vi "UI-main.vi"() -> ()   [LabVIEW 2013]
uses:
  <vilib>/LabVIEW Targets/FPGA/cRIO/shared/nicrio_ModuleControls/nicrio_cRIO-9229_DataRatesRing.ctl
  <vilib>/LabVIEW Targets/FPGA/cRIO/shared/nicrio_ModuleControls/nicrio_cRIO-9205_VoltageRange.ctl
  <vilib>/LabVIEW Targets/FPGA/cRIO/shared/nicrio_ModuleControls/nicrio_cRIO-9205_TerminalMode.ctl
panel:
  in  "配置簇":T4={"9205Count(uSec)"=1000, "9229采样率"=25, "update9213"=TRUE, "9213转换时间"=enum."High Speed", "9205Update AI Setings"=TRUE, "9205AI Channel Settings"=[{"Voltage Range"=enum."+/- 10V", "Terminal Mode"=enum."RSE"}, {"Voltage Range"=enum."+/- 10V", "Terminal Mode"=enum."RSE"}, {"Voltage Range"=enum."+/- 10V", "Terminal Mode"=enum."RSE"}, {"Voltage Range"=enum."+/- 10V", "Terminal Mode"=enum."RSE"}, {"Voltage Range"=enum."+/- 10V", "Terminal Mode"=enum."RSE"}, {"Voltage Range"=enum."+/- 10V", "Terminal Mode"=enum."RSE"}, {"Voltage Range"=enum."+/- 10V", "Terminal Mode"=enum."RSE"}, {"Voltage Range"=enum."+/- 10V", "Terminal Mode"=enum."RSE"}, {"Voltage Range"=enum."+/- 10V", "Terminal Mode"=enum."RSE"}, {"Voltage Range"=enum."+/- 10V", "Terminal Mode"=enum."RSE"}, {"Voltage Range"=enum."+/- 10V", "Terminal Mode"=enum."RSE"}, {"Voltage Range"=enum."+/- 10V", "Terminal Mode"=enum."RSE"}, {"Voltage Range"=enum."+/- 10V", "Terminal Mode"=enum."RSE"}, {"Voltage Range"=enum."+/- 10V", "Terminal Mode"=enum."RSE"}, {"Voltage Range"=enum."+/- 10V", "Terminal Mode"=enum."RSE"}, {"Voltage Range"=enum."+/- 10V", "Terminal Mode"=enum."RSE"}, {"Voltage Range"=enum."+/- 10V", "Terminal Mode"=enum."RSE"}, {"Voltage Range"=enum."+/- 10V", "Terminal Mode"=enum."RSE"}, {"Voltage Range"=enum."+/- 10V", "Terminal Mode"=enum."RSE"}, {"Voltage Range"=enum."+/- 10V", "Terminal Mode"=enum."RSE"}, {"Voltage Range"=enum."+/- 10V", "Terminal Mode"=enum."RSE"}, {"Voltage Range"=enum."+/- 10V", "Terminal Mode"=enum."RSE"}, {"Voltage Range"=enum."+/- 10V", "Terminal Mode"=enum."RSE"}, {"Voltage Range"=enum."+/- 10V", "Terminal Mode"=enum."RSE"}, {"Voltage Range"=enum."+/- 10V", "Terminal Mode"=enum."RSE"}]} {"9229采样率" items=["", "50.000 kS/s (NI 9229)", "25.000 kS/s (NI 9229)", "16.667 kS/s (NI 9229)", "12.500 kS/s (NI 9229)", "10.000 kS/s (NI 9229)", "8.333 kS/s (NI 9229)", "7.143 kS/s (NI 9229)", "6.250 kS/s (NI 9229)", "5.556 kS/s (NI 9229)", "5.000 kS/s (NI 9229)", "4.545 kS/s (NI 9229)", "4.167 kS/s (NI 9229)", "3.846 kS/s (NI 9229)", "3.571 kS/s (NI 9229)", "3.333 kS/s (NI 9229)", "3.125 kS/s (NI 9229)", "2.941 kS/s (NI 9229)", "2.778 kS/s (NI 9229)", "2.632 kS/s (NI 9229)", "2.500 kS/s (NI 9229)", "2.381 kS/s (NI 9229)", "2.273 kS/s (NI 9229)", "2.174 kS/s (NI 9229)", "2.083 kS/s (NI 9229)", "2.000 kS/s (NI 9229)", "1.923 kS/s (NI 9229)", "1.852 kS/s (NI 9229)", "1.786 kS/s (NI 9229)", "1.724 kS/s (NI 9229)", "1.667 kS/s (NI 9229)", "1.613 kS/s (NI 9229)"]}
  in  "选项卡控件":T5(tab)=enum."9205电流监控 "
  out "9213数据":T6(graph)={1372.0, 1372.0, 0.0, 0.0, 0.0, 0.0, 0.0, 0.0, 0.0, 0.0, 0.0, 0.0, 0.0, 0.0, 0.0, 0.0}
  out "9213通道1数据":dbl=1372.0
  out "9213通道2数据":dbl=1372.0
  out "9213通道3数据":dbl
  out "9213通道4数据":dbl
  out "9213通道5数据":dbl
  out "9213通道6数据":dbl
  out "9213通道7数据":dbl
  out "9213通道8数据":dbl
  out "9213通道9数据":dbl
  out "9213通道10数据":dbl
  out "9213通道11数据":dbl
  out "9213通道12数据":dbl
  out "9213通道13数据":dbl
  out "9213通道14数据":dbl
  out "9213通道15数据":dbl
  out "9213通道16数据":dbl
  out "9229通道12数据":dbl
  out "9229通道8数据":dbl
  out "9229通道10数据":dbl
  out "9229通道9数据":dbl
  out "9229通道6数据":dbl
  out "9229通道5数据":dbl
  out "9229通道4数据":dbl
  out "9229通道3数据":dbl
  out "9229通道2数据":dbl=24.32616424560547
  out "9229通道1数据":dbl=0.00066375732421875
  out "9229通道7数据":dbl
  out "9229通道11数据":dbl
  out "9229通道13数据":dbl
  out "9229通道14数据":dbl
  out "9229通道15数据":dbl
  out "9229通道16数据":dbl
  out "9229":T6(graph)={0.00066375732421875, 24.32616424560547, 0.0, 0.0, 0.0, 0.0, 0.0, 0.0, 0.0, 0.0, 0.0, 0.0, 0.0, 0.0, 0.0, 0.0}
  out "9205电压通道2":dbl=-3.0960659980773926
  out "9205电压通道1":dbl=-3.097379207611084
  out "9205电压通道3":dbl
  out "9205电压通道4":dbl
  out "9205电压通道5":dbl
  out "9205电压通道6":dbl
  out "9205电压通道7":dbl
  out "9205电压通道8":dbl
  out "9205电压通道9":dbl
  out "9205电压通道10":dbl
  out "9205电压通道11":dbl
  out "9205电压通道12":dbl
  out "9205电压通道13":dbl
  out "9205电压通道14":dbl
  out "9205电压通道15":dbl
  out "9205电压通道16":dbl
  out "9205电压通道17":dbl
  out "9205电压通道18":dbl
  out "9205电压通道19":dbl
  out "9205电压通道20":dbl
  out "9205电压通道21":dbl
  out "9205电压通道22":dbl
  out "9205电压通道23":dbl
  out "9205电压通道24":dbl
  out "9205电压":T7(graph)={-3.097379207611084, -3.0960659980773926, 0.0, 0.0, 0.0, 0.0, 0.0, 0.0, 0.0, 0.0, 0.0, 0.0, 0.0, 0.0, 0.0, 0.0, 0.0, 0.0, 0.0, 0.0, 0.0, 0.0, 0.0, 0.0, 0.0}
  out "9205电压通道25":dbl
  out "9205电流通道2":dbl=-3.0373048782348633
  out "9205电流通道1":dbl=-3.005133628845215
  out "9205电流通道3":dbl
  out "9205电流通道4":dbl
  out "9205电流通道5":dbl
  out "9205电流通道6":dbl
  out "9205电流通道7":dbl
  out "9205电流 2":cluster{dbl, dbl, dbl, dbl, dbl, dbl, dbl}(graph)={-3.005133628845215, -3.0373048782348633, 0.0, 0.0, 0.0, 0.0, 0.0}
  in  "9205电流":string(tree)="2"
  in  "9205电压":string(tree)="2"
  in  "9213温度":string(tree)="2"
  in  "9229电压":string(tree)="2"
  out "连接成功？":bool
  out "UI命令":string="退出"
  in  "停止发送数据到UI":bool
  in  "发送数据到UI":bool
  in  "连接":bool=TRUE
  in  "触发采集":bool=TRUE
  in  "退出":bool=TRUE
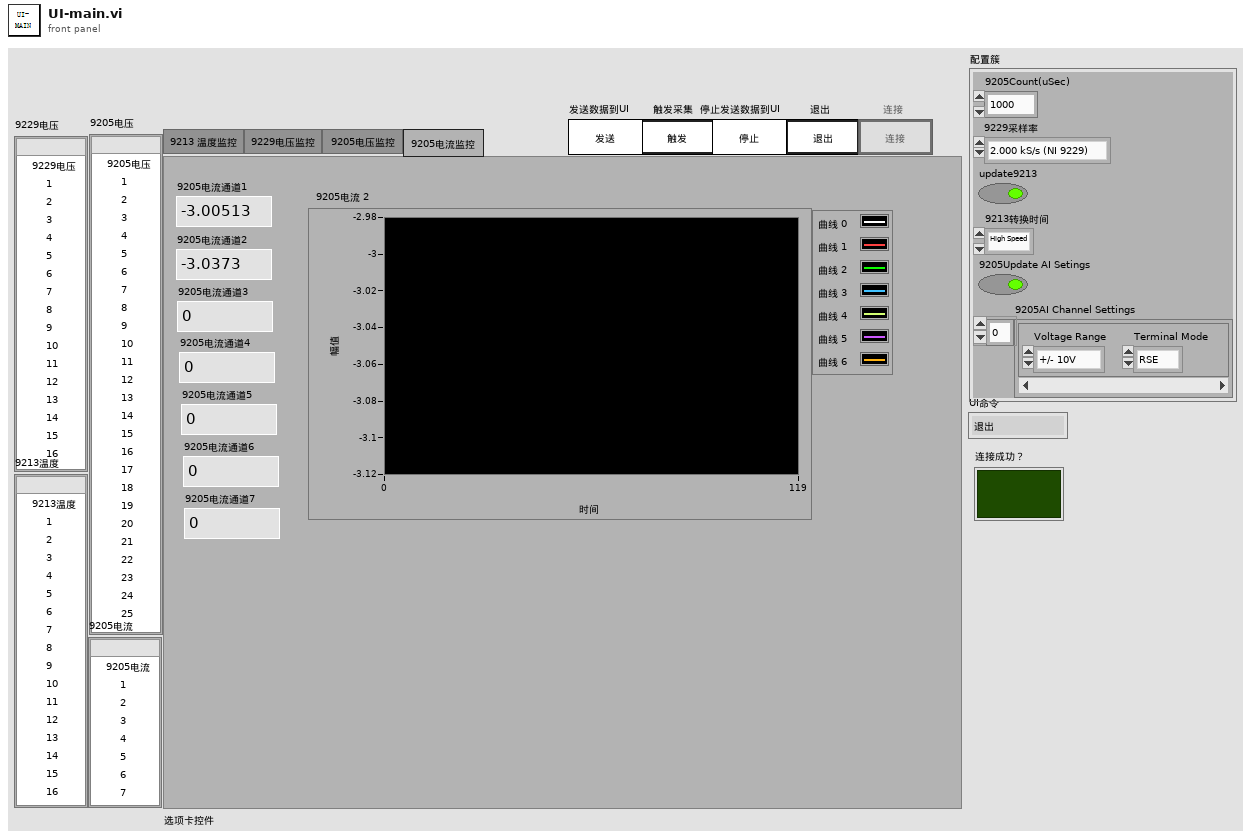
[diagram p1: front panel]
types:
  T1 = typedef "nicrio_cRIO-9229_DataRatesRing.ctl" = u8
  T2 = typedef "nicrio_cRIO-9205_VoltageRange.ctl" = enum8{"+/- 10V", "+/- 5V", "+/- 1V", "+/- 200mV"}
  T3 = typedef "nicrio_cRIO-9205_TerminalMode.ctl" = enum8{"RSE", "NRSE", "DIFF"}
  T4 = cluster{"9205Count(uSec)":u32, "9229采样率":T1, "update9213":bool, "9213转换时间":enum8{"High Speed", "High Resolution"}, "9205Update AI Setings":bool, "9205AI Channel Settings":cluster{"Voltage Range":T2, "Terminal Mode":T3}[]}
  T5 = enum32{"9213 温度监控", "9229电压监控", "9205电压监控 ", "9205电流监控 "}
  T6 = cluster{dbl, dbl, dbl, dbl, dbl, dbl, dbl, dbl, dbl, dbl, dbl, dbl, dbl, dbl, dbl, dbl}
  T7 = cluster{dbl, dbl, dbl, dbl, dbl, dbl, dbl, dbl, dbl, dbl, dbl, dbl, dbl, dbl, dbl, dbl, dbl, dbl, dbl, dbl, dbl, dbl, dbl, dbl, dbl}
  T8 = enum16{"open", "open or create", "create or replace", "create", "open (read-only)"}
  T9 = typedef "消息命令控件.ctl" = cluster{"message":string, "变体数据":variant}
  T10 = typedef "LVPoint32TypeDef.ctl" = cluster{"Horizontal":i32, "Vertical":i32}
  T11 = enum8{"Enabled", "Disabled", "Disabled and Grayed Out"}
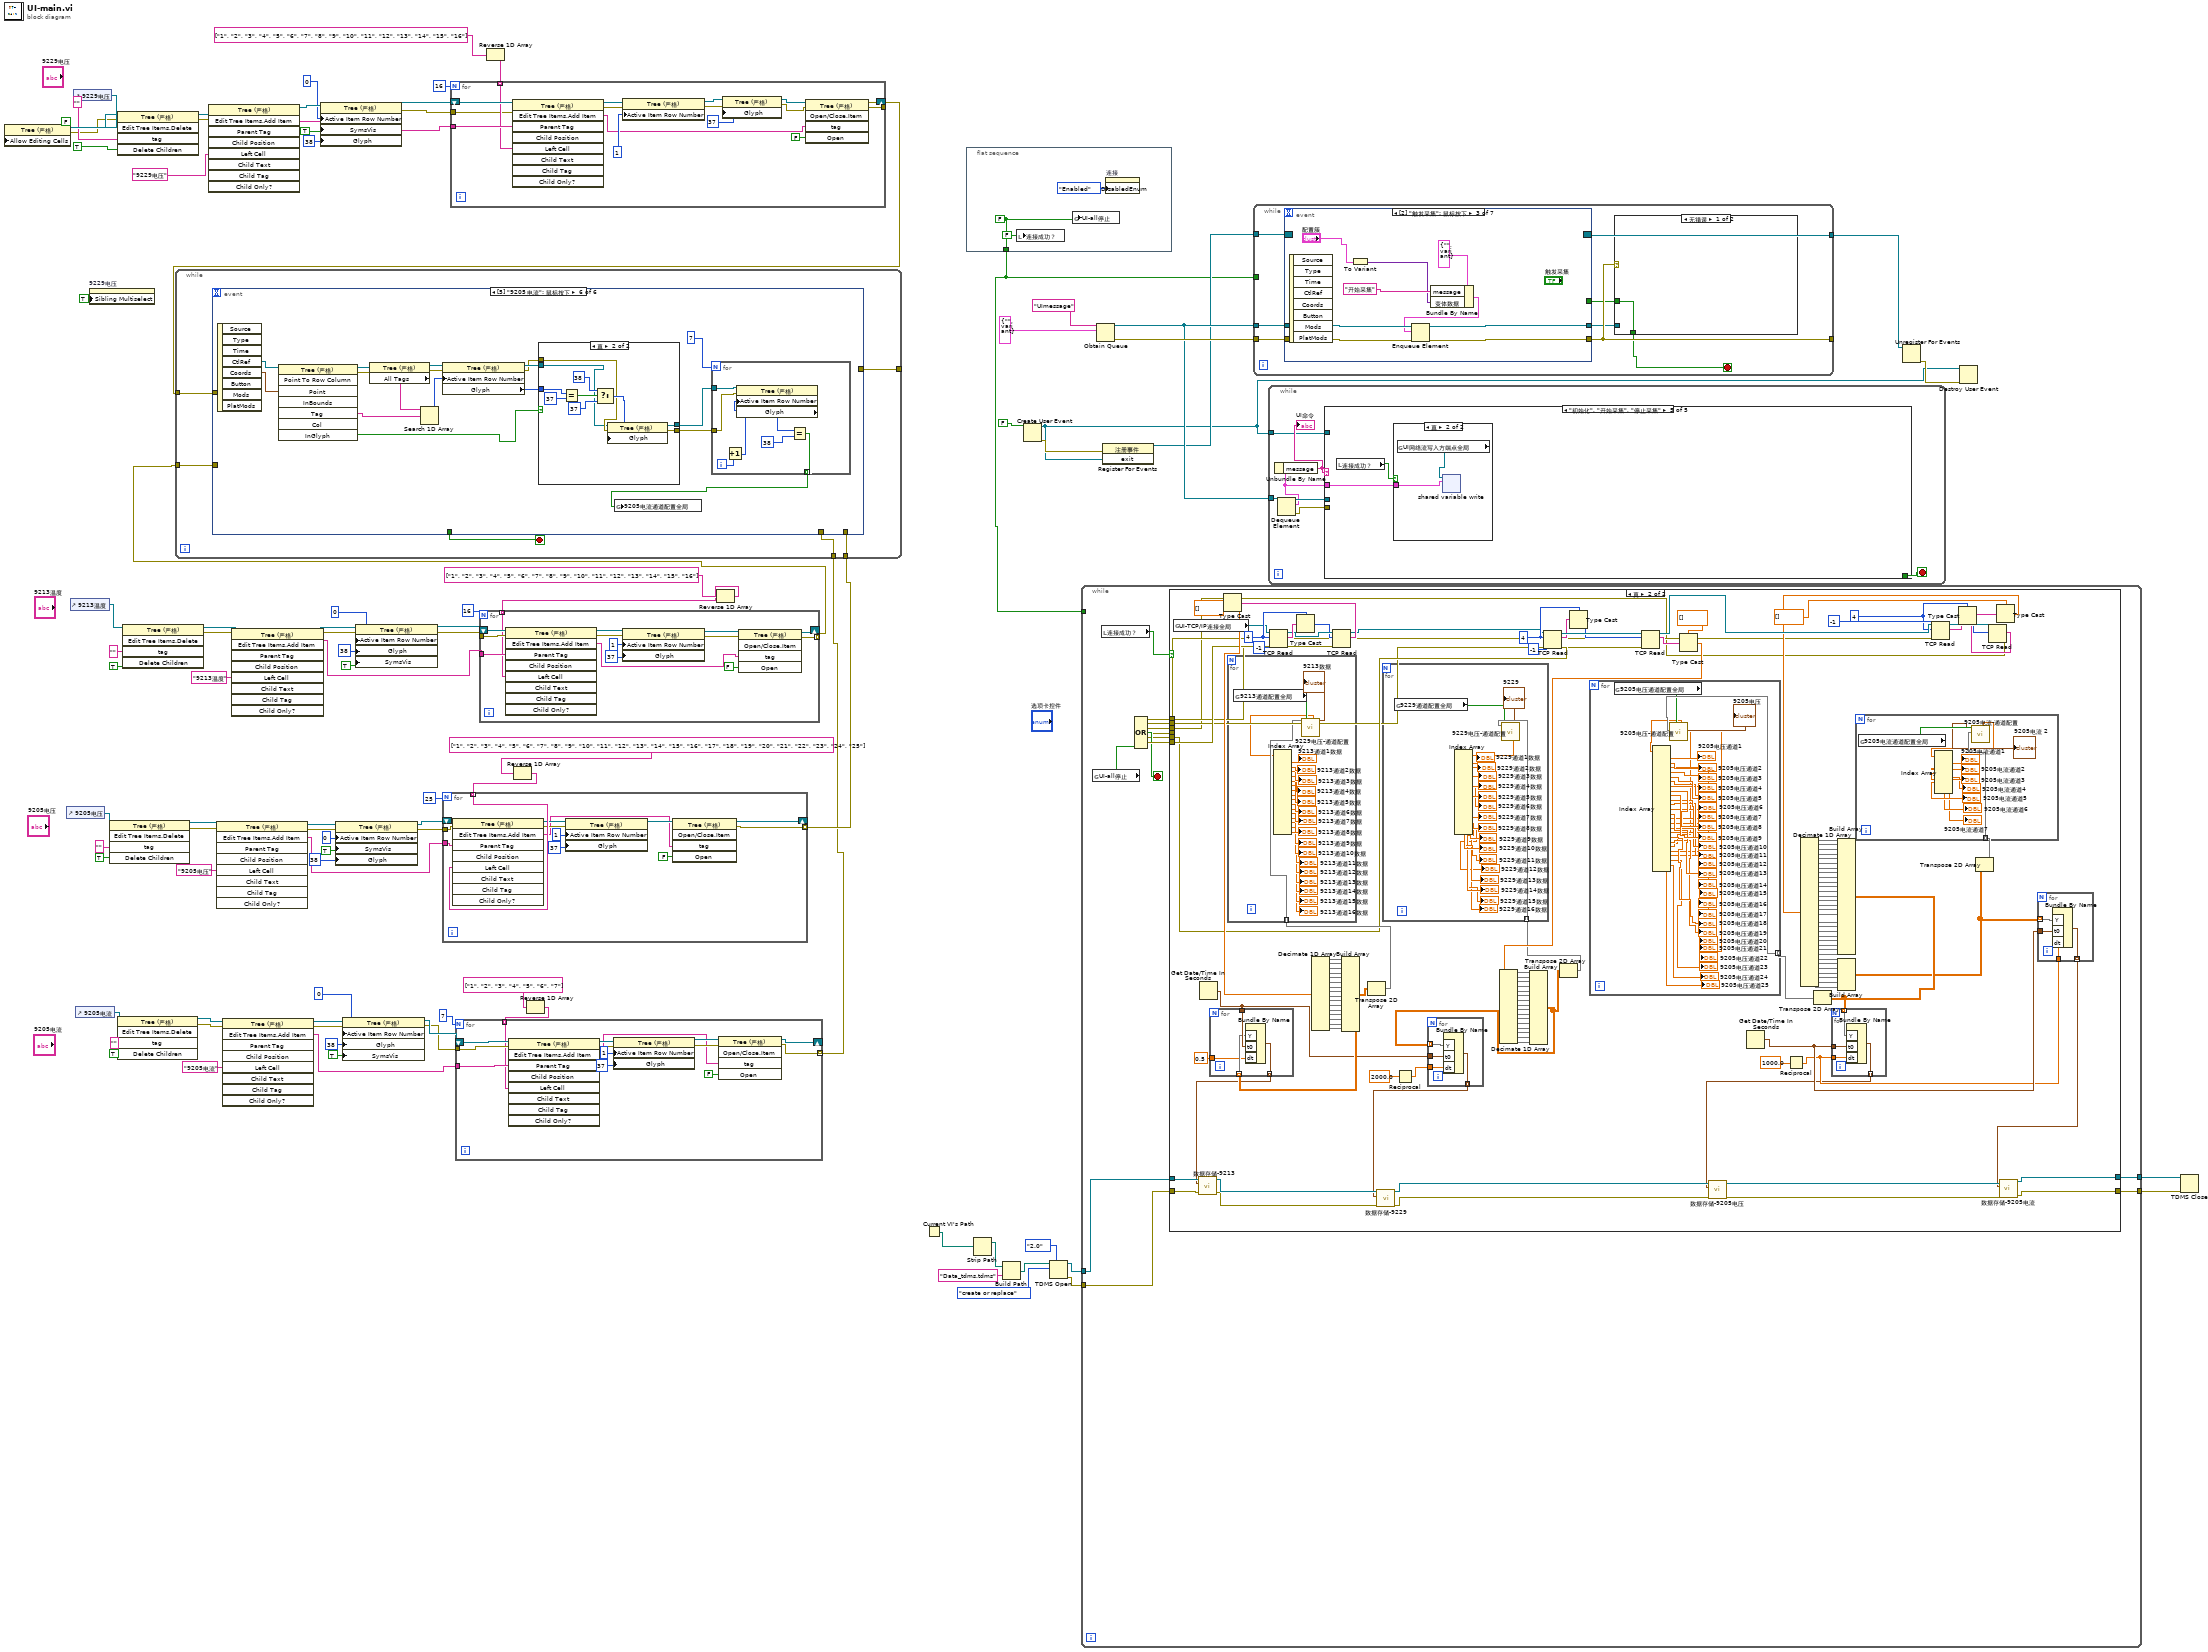
[diagram p0: block diagram]
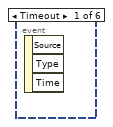
[diagram p2: hidden frame]
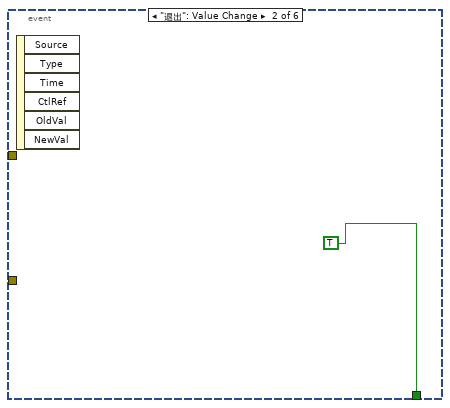
[diagram p3: hidden frame]
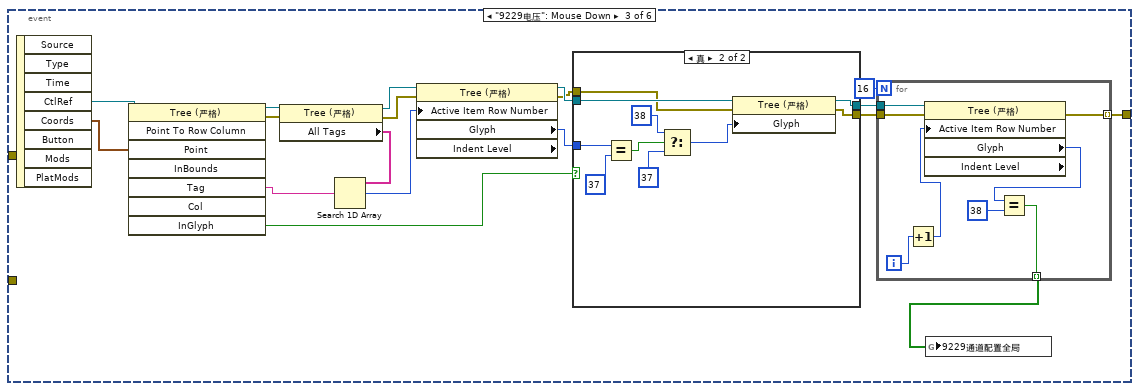
[diagram p4: hidden frame]
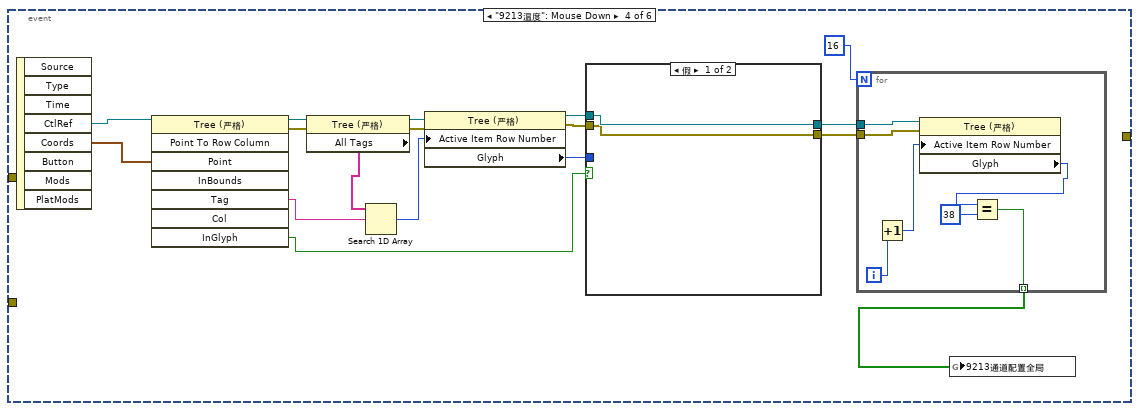
[diagram p6: hidden frame]
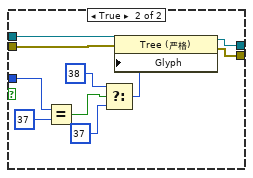
[diagram p7: hidden frame]
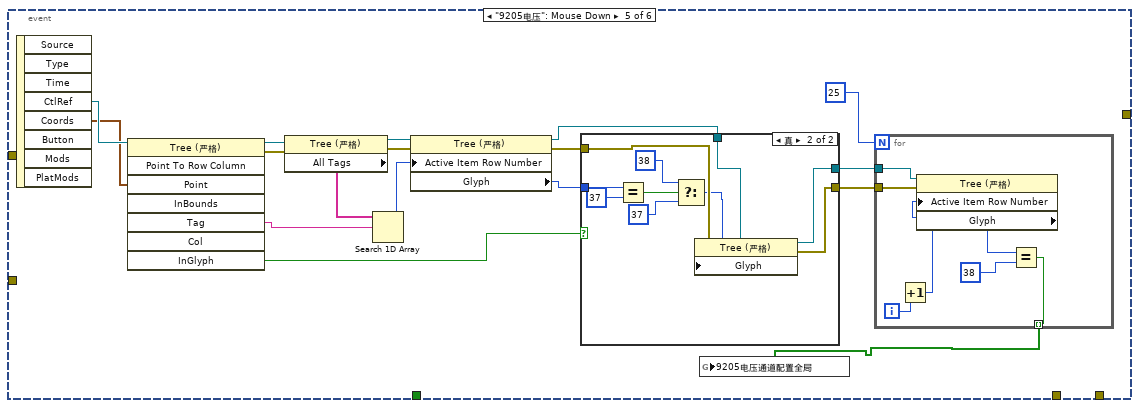
[diagram p8: hidden frame]
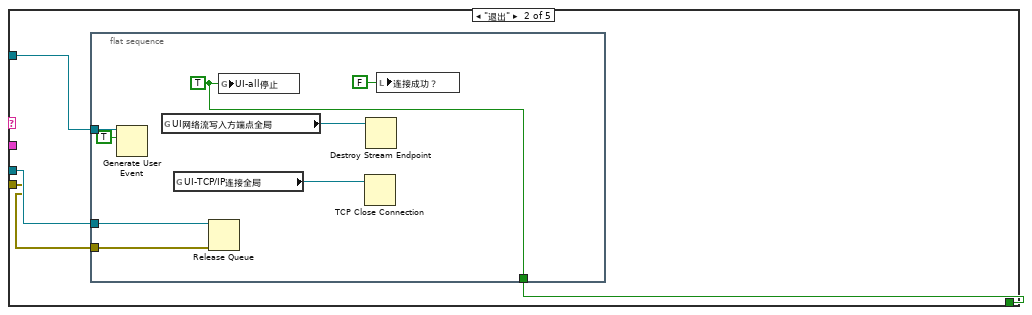
[diagram p13: hidden frame]
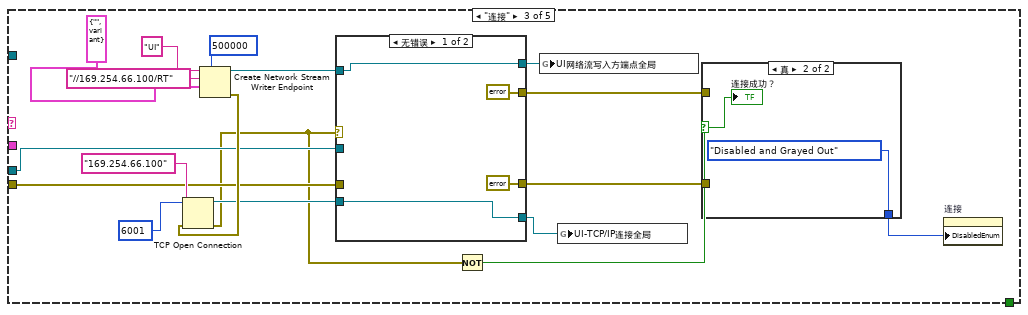
[diagram p14: hidden frame]
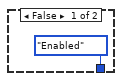
[diagram p15: hidden frame]
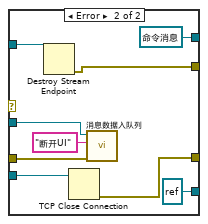
[diagram p16: hidden frame]
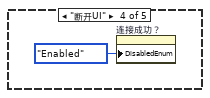
[diagram p17: hidden frame]
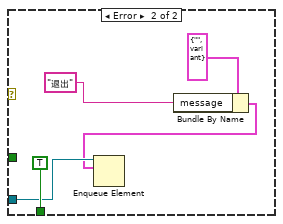
[diagram p19: hidden frame]
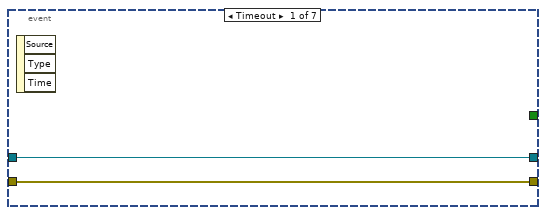
[diagram p20: hidden frame]
diagram:
  n1 = control-ref of="9205电压"() -> (w53:refnum<vi>)
  n2 = control-ref of="9213温度"() -> (w71:refnum<vi>)
  n3 = control-ref of="9229电压"() -> (w91:refnum<vi>)
  n4 = property class="Tree (严格)"(reference=w91, "Allow Editing Cells"=FALSE ("允许编辑单元格")) -> (reference out=w89:refnum<vi>, error out=w84:errorcluster)  [unwired: 1 in]
  n5 = control-ref of="9205电流"() -> (w37:refnum<vi>)
  n6 = property on="9229电压" class="Tree (严格)"("Sibling Multiselect"=TRUE ("同辈多选")) -> ()  [unwired: 2 in, 2 out]
  n7 = invoke class="Tree (严格)" method="Edit Tree Items.Delete"(reference=w53, "tag"="" ("标识符"), "Delete Children"=TRUE ("删除子项？")) -> (reference out=w50:refnum<vi>, error out=w49:errorcluster)  [unwired: 2 in, 3 out]
  n8 = invoke class="Tree (严格)" method="Edit Tree Items.Delete"(reference=w37, "tag"="" ("标识符"), "Delete Children"=TRUE ("删除子项？")) -> (reference out=w34:refnum<vi>, error out=w33:errorcluster)  [unwired: 2 in, 3 out]
  n9 = invoke class="Tree (严格)" method="Edit Tree Items.Delete"(reference=w89, error in=w84, "tag"="" ("标识符"), "Delete Children"=TRUE ("删除子项？")) -> (reference out=w87:refnum<vi>, error out=w83:errorcluster)  [unwired: 1 in, 3 out]
  n10 = invoke class="Tree (严格)" method="Edit Tree Items.Delete"(reference=w71, "tag"="" ("标识符"), "Delete Children"=TRUE ("删除子项？")) -> (reference out=w68:refnum<vi>, error out=w67:errorcluster)  [unwired: 2 in, 3 out]
  n11 = invoke class="Tree (严格)" method="Edit Tree Items.Add Item"(reference=w87, error in=w83, "Left Cell"="9229电压" ("左单元格字符串")) -> (reference out=w81:refnum<vi>, "Edit Tree Items:Add Item"=w73:string)  [unwired: 6 in, 7 out]
  n12 = invoke class="Tree (严格)" method="Edit Tree Items.Add Item"(reference=w50, error in=w49, "Left Cell"="9205电压" ("左单元格字符串")) -> (reference out=w47:refnum<vi>, error out=w46:errorcluster, "Edit Tree Items:Add Item"=w41:string)  [unwired: 6 in, 6 out]
  n13 = invoke class="Tree (严格)" method="Edit Tree Items.Add Item"(reference=w34, error in=w33, "Left Cell"="9205电流" ("左单元格字符串")) -> (reference out=w31:refnum<vi>, error out=w30:errorcluster, "Edit Tree Items:Add Item"=w22:string)  [unwired: 6 in, 6 out]
  n14 = invoke class="Tree (严格)" method="Edit Tree Items.Add Item"(reference=w68, error in=w67, "Left Cell"="9213温度" ("左单元格字符串")) -> (reference out=w65:refnum<vi>, error out=w64:errorcluster, "Edit Tree Items:Add Item"=w56:string)  [unwired: 6 in, 6 out]
  n15 = property class="Tree (严格)"(reference=w81, "Active Item Row Number"=0 ("活动项:行数"), "SymsVis"=TRUE ("显示项:显示符号"), "Glyph"=38 ("活动项:符号索引")) -> (reference out=w77:refnum<vi>, error out=w76:errorcluster)  [unwired: 1 in]
  n16 = property class="Tree (严格)"(reference=w47, error in=w46, "Active Item Row Number"=0 ("活动项:行数"), "SymsVis"=TRUE ("显示项:显示符号"), "Glyph"=38 ("活动项:符号索引")) -> (reference out=w43:refnum<vi>, error out=w42:errorcluster)
  n17 = property class="Tree (严格)"(reference=w31, error in=w30, "Active Item Row Number"=0 ("活动项:行数"), "Glyph"=38 ("活动项:符号索引"), "SymsVis"=TRUE ("显示项:显示符号")) -> (reference out=w24:refnum<vi>, error out=w23:errorcluster)
  n18 = property class="Tree (严格)"(reference=w65, error in=w64, "Active Item Row Number"=0 ("活动项:行数"), "Glyph"=38 ("活动项:符号索引"), "SymsVis"=TRUE ("显示项:显示符号")) -> (reference out=w58:refnum<vi>, error out=w57:errorcluster)
  n19 = Reverse 1D Array(array=string[] ["1", "2", "3", "4", "5", "6", "7", "8", "9", "10", "11", "12", "13", "14", "15", "16"]) -> (reversed array=w79:string[])
  n20 = for {
    N: 16 -> [_]
    tunnel: w73 -> [w112]
    tunnel: w79 -> [w110] mode=indexing
    tunnel: w76 -> [w109]
    tunnel: [w103] -> w72
    shift-right: [w102] -> _
    shift-left: w77 -> [w111]
    n21 = invoke class="Tree (严格)" method="Edit Tree Items.Add Item"(reference=w111, error in=w109, "Parent Tag"=w112, "Left Cell"=w110) -> (reference out=w108:refnum<vi>, error out=w107:errorcluster, "Edit Tree Items:Add Item"=w98:string)  [unwired: 5 in, 6 out]
    n22 = property class="Tree (严格)"(reference=w108, error in=w107, "Active Item Row Number"=1 ("活动项:行数")) -> (reference out=w106:refnum<vi>, error out=w99:errorcluster)
    n23 = property class="Tree (严格)"(reference=w106, error in=w99, "Glyph"=37 ("活动项:符号索引")) -> (reference out=w101:refnum<vi>, error out=w100:errorcluster)
    n24 = invoke class="Tree (严格)" method="Open/Close.Item"(reference=w101, error in=w100, "tag"=w98, "Open"=FALSE ("打开？")) -> (reference out=w102:refnum<vi>, error out=w103:errorcluster)  [unwired: 1 in, 3 out]
  }
  n25 = Reverse 1D Array(array=string[] ["1", "2", "3", "4", "5", "6", "7", "8", "9", "10", "11", "12", "13", "14", "15", "16", "17", "18", "19", "20", "21", "22", "23", "24", "25"]) -> (reversed array=w39:string[])
  n26 = for {
    N: 25 -> [_]
    tunnel: w42 -> [w124]
    shift-right: [w116] -> _
    shift-left: w43 -> [w125]
    tunnel: w41 -> [w123]
    tunnel: w39 -> [w122] mode=indexing
    tunnel: [w113] -> w38 mode=indexing
    n27 = invoke class="Tree (严格)" method="Edit Tree Items.Add Item"(reference=w125, error in=w124, "Parent Tag"=w123, "Left Cell"=w122) -> (reference out=w121:refnum<vi>, error out=w120:errorcluster, "Edit Tree Items:Add Item"=w115:string)  [unwired: 5 in, 6 out]
    n28 = property class="Tree (严格)"(reference=w121, error in=w120, "Active Item Row Number"=1 ("活动项:行数"), "Glyph"=37 ("活动项:符号索引")) -> (reference out=w117:refnum<vi>)  [unwired: 1 out]
    n29 = invoke class="Tree (严格)" method="Open/Close.Item"(reference=w117, "tag"=w115, "Open"=FALSE ("打开？")) -> (reference out=w116:refnum<vi>, error out=w113:errorcluster)  [unwired: 2 in, 3 out]
  }
  n30 = Reverse 1D Array(array=string[] ["1", "2", "3", "4", "5", "6", "7"]) -> (reversed array=w20:string[])
  n31 = for {
    N: 7 -> [_]
    shift-right: [w127] -> _
    shift-left: w24 -> [w139]
    tunnel: w23 -> [w138]
    tunnel: w22 -> [w137]
    tunnel: w20 -> [w136] mode=indexing
    tunnel: [w126] -> w19 mode=indexing
    n32 = invoke class="Tree (严格)" method="Edit Tree Items.Add Item"(reference=w139, error in=w138, "Parent Tag"=w137, "Left Cell"=w136) -> (reference out=w135:refnum<vi>, error out=w134:errorcluster, "Edit Tree Items:Add Item"=w129:string)  [unwired: 5 in, 6 out]
    n33 = property class="Tree (严格)"(reference=w135, error in=w134, "Active Item Row Number"=1 ("活动项:行数"), "Glyph"=37 ("活动项:符号索引")) -> (reference out=w131:refnum<vi>, error out=w130:errorcluster)
    n34 = invoke class="Tree (严格)" method="Open/Close.Item"(reference=w131, error in=w130, "tag"=w129, "Open"=FALSE ("打开？")) -> (reference out=w127:refnum<vi>, error out=w126:errorcluster)  [unwired: 1 in, 3 out]
  }
  n35 = Reverse 1D Array(array=string[] ["1", "2", "3", "4", "5", "6", "7", "8", "9", "10", "11", "12", "13", "14", "15", "16"]) -> (reversed array=w55:string[])
  n36 = for {
    N: 16 -> [_]
    tunnel: w57 -> [w152]
    shift-right: [w141] -> _
    shift-left: w58 -> [w153]
    tunnel: w56 -> [w151]
    tunnel: w55 -> [w150] mode=indexing
    tunnel: [w140] -> w54 mode=indexing
    n37 = invoke class="Tree (严格)" method="Edit Tree Items.Add Item"(reference=w153, error in=w152, "Parent Tag"=w151, "Left Cell"=w150) -> (reference out=w149:refnum<vi>, error out=w148:errorcluster, "Edit Tree Items:Add Item"=w143:string)  [unwired: 5 in, 6 out]
    n38 = property class="Tree (严格)"(reference=w149, error in=w148, "Active Item Row Number"=1 ("活动项:行数"), "Glyph"=37 ("活动项:符号索引")) -> (reference out=w145:refnum<vi>, error out=w144:errorcluster)
    n39 = invoke class="Tree (严格)" method="Open/Close.Item"(reference=w145, error in=w144, "tag"=w143, "Open"=FALSE ("打开？")) -> (reference out=w141:refnum<vi>, error out=w140:errorcluster)  [unwired: 1 in, 3 out]
  }
  n40 = while {
    tunnel: w72 -> [w158]
    tunnel: [w157] -> _
    tunnel: w54 -> [w156]
    tunnel: w38 -> [w155]
    tunnel: w19 -> [w154]
    stop <- w159 stop-if-true
    n41 = event shown="[5] \"9205电流\": 鼠标按下" {
      selector: _ -> [_ _ _ _ _ _]
      dyn-events: _ -> [_ _ _ _ _ _]
      timeout: _ -> [_ _ _ _ _ _]
      tunnel: [_ TRUE ("停止") _ _ _ _] -> w159
      tunnel: w158 -> [_ _ _ _ _ _]
      tunnel: [_ _ w162 _ _ _] -> w157
      tunnel: w156 -> [_ _ _ _ _ _]
      tunnel: w155 -> [_ _ _ _ _ _]
      tunnel: w154 -> [_ _ _ _ _ _]
      event Timeout {
        n42 = event-data() -> ()  [unwired: 1 in, 3 out]
      }
      event "退出": Value Change {
        n43 = event-data() -> ()  [unwired: 1 in, 6 out]
      }
      event "9229电压": Mouse Down {
        n44 = event-data() -> ("CtlRef"=w166:refnum<vi>, "Coords"=w178:T10)  [unwired: 1 in, 6 out]
        n45 = invoke class="Tree (严格)" method="Point To Row Column"(reference=w166, "Point"=w178) -> (reference out=w177:refnum<vi>, error out=w172:errorcluster, "Tag"=w175:string, "InGlyph"=w173:bool)  [unwired: 6 in, 4 out]
        n46 = property class="Tree (严格)"(reference=w177, error in=w172) -> (reference out=w174:refnum<vi>, error out=w171:errorcluster, "All Tags"=w176:string[])
        n47 = Search 1D Array(1D array=w176, element=w175) -> (index of element=w167:i32)  [unwired: 1 in]
        n48 = property class="Tree (严格)" props=["Active Item Row Number", "Glyph", "Indent Level"](reference=w174, error in=w171, "Active Item Row Number"=w167) -> (reference out=w169:refnum<vi>, error out=w168:errorcluster, "Glyph"=w170:i32)  [unwired: 1 out]
        n49 = case shown="真" w173 {
          tunnel: w170 -> [_ w198]
          tunnel: w169 -> [w187 w194]
          tunnel: w168 -> [w188 w193]
          tunnel: [w188 w190] -> w164
          tunnel: [w187 w189] -> w163
          frame False {
          }
          frame True {
            n50 = Equal?(x=w198, y=37) -> (x = y?=w191:bool)
            n51 = Select(t=38 ("y"), s=w191, f=37 ("y")) -> (s? t:f=w192:i32)
            n52 = property class="Tree (严格)"(reference=w194, error in=w193, "Glyph"=w192) -> (reference out=w189:refnum<vi>, error out=w190:errorcluster)
          }
        }
        n53 = for {
          N: 16 -> [_]
          tunnel: w164 -> [w184]
          tunnel: w163 -> [w183]
          tunnel: [w180] -> w161 mode=indexing
          tunnel: [w179] -> w162 mode=indexing
          i -> [w186]
          n54 = Increment(x=w186) -> (x+1=w185:i32)
          n55 = property class="Tree (严格)" props=["Active Item Row Number", "Glyph", "Indent Level"](reference=w183, error in=w184, "Active Item Row Number"=w185) -> (error out=w179:errorcluster, "Glyph"=w182:i32)  [unwired: 2 out]
          n56 = Equal?(x=w182, y=38) -> (x = y?=w180:bool)
        }
        n57 = global write "9229通道配置全局.vi" "9229通道配置全局"(w161) -> ()
      }
      event "9213温度": Mouse Down {
        n58 = event-data() -> ("CtlRef"=w215:refnum<vi>, "Coords"=w214:T10)  [unwired: 1 in, 6 out]
        n59 = invoke class="Tree (严格)" method="Point To Row Column"(reference=w215, "Point"=w214) -> (reference out=w212:refnum<vi>, error out=w211:errorcluster, "Tag"=w213:string, "InGlyph"=w206:bool)  [unwired: 6 in, 4 out]
        n60 = property class="Tree (严格)"(reference=w212, error in=w211) -> (reference out=w209:refnum<vi>, error out=w208:errorcluster, "All Tags"=w210:string[])
        n61 = Search 1D Array(1D array=w210, element=w213) -> (index of element=w207:i32)  [unwired: 1 in]
        n62 = property class="Tree (严格)"(reference=w209, error in=w208, "Active Item Row Number"=w207) -> (reference out=w204:refnum<vi>, error out=w203:errorcluster, "Glyph"=w205:i32)
        n63 = case shown="假" w206 {
          tunnel: w205 -> [_ w234]
          tunnel: w204 -> [w224 w229]
          tunnel: w203 -> [w223 w228]
          tunnel: [w224 w226] -> w201
          tunnel: [w223 w225] -> w200
          frame False {
          }
          frame True {
            n64 = Equal?(x=w234, y=37) -> (x = y?=w232:bool)
            n65 = Select(t=38 ("y"), s=w232, f=37 ("y")) -> (s? t:f=w227:i32)
            n66 = property class="Tree (严格)"(reference=w229, error in=w228, "Glyph"=w227) -> (reference out=w226:refnum<vi>, error out=w225:errorcluster)
          }
        }
        n67 = for {
          N: 16 -> [_]
          tunnel: w201 -> [w222]
          tunnel: w200 -> [w221]
          tunnel: [w216] -> w199 mode=indexing
          i -> [w220]
          n68 = Increment(x=w220) -> (x+1=w219:i32)
          n69 = property class="Tree (严格)"(reference=w222, error in=w221, "Active Item Row Number"=w219) -> ("Glyph"=w218:i32)  [unwired: 2 out]
          n70 = Equal?(x=w218, y=38) -> (x = y?=w216:bool)
        }
        n71 = global write "9213通道配置全局.vi" "9213通道配置全局"(w199) -> ()
      }
      event "9205电压": Mouse Down {
        n72 = event-data() -> ("CtlRef"=w251:refnum<vi>, "Coords"=w250:T10)  [unwired: 1 in, 6 out]
        n73 = invoke class="Tree (严格)" method="Point To Row Column"(reference=w251, "Point"=w250) -> (reference out=w249:refnum<vi>, error out=w248:errorcluster, "Tag"=w246:string, "InGlyph"=w245:bool)  [unwired: 6 in, 4 out]
        n74 = property class="Tree (严格)"(reference=w249, error in=w248) -> (reference out=w244:refnum<vi>, error out=w243:errorcluster, "All Tags"=w247:string[])
        n75 = Search 1D Array(1D array=w247, element=w246) -> (index of element=w242:i32)  [unwired: 1 in]
        n76 = property class="Tree (严格)"(reference=w244, error in=w243, "Active Item Row Number"=w242) -> (reference out=w240:refnum<vi>, error out=w239:errorcluster, "Glyph"=w241:i32)
        n77 = case shown="真" w245 {
          tunnel: w241 -> [_ w270]
          tunnel: w240 -> [w259 w265]
          tunnel: w239 -> [w260 w264]
          tunnel: [w259 w262] -> w237
          tunnel: [w260 w261] -> w236
          frame False {
          }
          frame True {
            n78 = Equal?(x=w270, y=37) -> (x = y?=w267:bool)
            n79 = Select(t=38 ("y"), s=w267, f=37 ("y")) -> (s? t:f=w263:i32)
            n80 = property class="Tree (严格)"(reference=w265, error in=w264, "Glyph"=w263) -> (reference out=w262:refnum<vi>, error out=w261:errorcluster)
          }
        }
        n81 = for {
          N: 25 -> [_]
          tunnel: w237 -> [w257]
          tunnel: w236 -> [w256]
          tunnel: [w252] -> w235 mode=indexing
          i -> [w258]
          n82 = Increment(x=w258) -> (x+1=w255:i32)
          n83 = property class="Tree (严格)"(reference=w257, error in=w256, "Active Item Row Number"=w255) -> ("Glyph"=w254:i32)  [unwired: 2 out]
          n84 = Equal?(x=w254, y=38) -> (x = y?=w252:bool)
        }
        n85 = global write "9205电压通道配置全局.vi" "9205电压通道配置全局"(w235) -> ()
      }
      event "9205电流": Mouse Down {
        n86 = event-data() -> ("CtlRef"=w279:refnum<vi>, "Coords"=w278:T10)  [unwired: 1 in, 6 out]
        n87 = invoke class="Tree (严格)" method="Point To Row Column"(reference=w279, "Point"=w278) -> (reference out=w287:refnum<vi>, error out=w286:errorcluster, "Tag"=w284:string, "InGlyph"=w277:bool)  [unwired: 6 in, 4 out]
        n88 = property class="Tree (严格)"(reference=w287, error in=w286) -> (reference out=w283:refnum<vi>, error out=w282:errorcluster, "All Tags"=w285:string[])
        n89 = Search 1D Array(1D array=w285, element=w284) -> (index of element=w281:i32)  [unwired: 1 in]
        n90 = property class="Tree (严格)"(reference=w283, error in=w282, "Active Item Row Number"=w281) -> (reference out=w276:refnum<vi>, error out=w275:errorcluster, "Glyph"=w274:i32)
        n91 = case shown="真" w277 {
          tunnel: w276 -> [w289 w292]
          tunnel: w275 -> [w288 w293]
          tunnel: w274 -> [_ w294]
          tunnel: [w289 w291] -> w273
          tunnel: [w288 w290] -> w272
          frame False {
          }
          frame True {
            n92 = Equal?(x=w294, y=37) -> (x = y?=w297:bool)
            n93 = Select(t=38 ("y"), s=w297, f=37 ("y")) -> (s? t:f=w295:i32)
            n94 = property class="Tree (严格)"(reference=w292, error in=w293, "Glyph"=w295) -> (reference out=w291:refnum<vi>, error out=w290:errorcluster)
          }
        }
        n95 = for {
          N: 7 -> [_]
          tunnel: [w302] -> w271 mode=indexing
          tunnel: w273 -> [w301]
          tunnel: w272 -> [w300]
          i -> [w306]
          n96 = Increment(x=w306) -> (x+1=w305:i32)
          n97 = property class="Tree (严格)"(reference=w301, error in=w300, "Active Item Row Number"=w305) -> ("Glyph"=w304:i32)  [unwired: 2 out]
          n98 = Equal?(x=w304, y=38) -> (x = y?=w302:bool)
        }
        n99 = global write "9205电流通道配置全局.vi" "9205电流通道配置全局"(w271) -> ()
      }
    }
  }
  n100 = Current VI's Path() -> (path=w12:path)
  n101 = flat-sequence {
    tunnel: [w307] -> w3
    frame #0 {
      w307 = FALSE ("UIdata停止")
      n102 = local write "连接成功？"(FALSE ("连接成功？")) -> ()
      n103 = global write "UI-all停止全局.vi" "UI-all停止"(w307) -> ()
      n104 = property on="连接" class="Bool"("DisabledEnum"=T11."Enabled" ("禁用")) -> ()  [unwired: 2 in, 2 out]
    }
  }
  n105 = Strip Path(path=w12) -> (stripped path=w13:path)  [unwired: 1 out]
  n106 = Build Path(base path=w13, name or relative path="Data_tdms.tdms" ("名称或相对路径")) -> (appended path=w15:path)
  n107 = Create User Event(user event datatype=FALSE ("exit")) -> (user event=w4:refnum<user-event>, error out=w7:errorcluster)  [unwired: 1 in]
  n108 = TDMS Open(7:enum16{"1.0", "2.0"}."2.0" ("文件格式版本(2.0)"), 10:T8."create or replace" ("操作(0:open)"), 11:w15) -> (0:w10:errorcluster, 3:w11:refnum<k34>)  [unwired: 4 in]
  n109 = while {
    tunnel: w11 -> [w322]
    tunnel: w10 -> [w321]
    tunnel: w3 -> [_]
    tunnel: [w314] -> w2
    tunnel: [w313] -> w1
    stop <- w317 stop-if-true
    n110 = global read "UI-all停止全局.vi" "UI-all停止"() -> (w319:bool)
    n111 = local read "连接成功？"() -> (w320:bool)
    n112 = case shown="真" w320 {
      tunnel: w322 -> [_ w344]
      tunnel: w321 -> [_ w343]
      tunnel: [_ w336] -> w318
      tunnel: [_ w335] -> w316
      tunnel: [_ w334] -> w315
      tunnel: [_ w327] -> w314
      tunnel: [_ w326] -> w313
      tunnel: [_ w325] -> w312
      tunnel: [_ w324] -> w311
      tunnel: [_ w323] -> w310
      frame False {
      }
      frame True {
        w430 = 4 ("读取的字节")
        w437 = 4 ("读取的字节")
        w444 = 4 ("读取的字节")
        n113 = global read "UI-TCP-IP连接全局.vi" "UI-TCP/IP连接全局"() -> (w345:refnum<k5>)
        n114 = Get Date/Time In Seconds() -> (seconds since 1Jan1904=w353:timestamp)
        n115 = TCP Read(connection ID=w345, bytes to read=w444, 9:-1 ("超时毫秒(25000)")) -> (connection ID out=w446:refnum<k5>, data out=w447:string, error out=w336:errorcluster)  [unwired: 2 in]
        n116 = Type Cast(type=w444, x=w447) -> (*(type *) &x=w443:i32)
        n117 = TCP Read(connection ID=w446, bytes to read=w443) -> (connection ID out=w346:refnum<k5>, data out=w445:string, error out=w325:errorcluster)  [unwired: 3 in]
        n118 = Type Cast(type=dbl[] [], x=w445) -> (*(type *) &x=w393:dbl[])
        n119 = Decimate 1D Array(w393) -> (w392:dbl[], w391:dbl[], w390:dbl[], w389:dbl[], w388:dbl[], w387:dbl[], w386:dbl[], w385:dbl[], w384:dbl[], w383:dbl[], w382:dbl[], w381:dbl[], w380:dbl[], w379:dbl[], w378:dbl[], w377:dbl[])
        n120 = Build Array(w392, w391, w390, w389, w388, w387, w386, w385, w384, w383, w382, w381, w380, w379, w378, w377) -> (w355:dbl[][])
        n121 = for {
          tunnel: [w464] -> w331 mode=indexing
          tunnel: w353 -> [w463]
          tunnel: w355 -> [w462] mode=indexing
          tunnel: 0.5 ("dt") -> [w461]
          n122 = Bundle By Name("Y"=w462, "t0"=w463, "dt"=w461) -> (w464:waveform(dbl))  [unwired: 1 in]
        }
        n123 = call "数据存储-9213.vi"("错误输入（无错误）"=w343, "9213数据"=w331, "tdms文件输入"=w344) -> ("错误输出"=w341:errorcluster, "tdms文件输出"=w342:refnum<k34>)  [unwired: 7 in]
        n124 = Transpose 2D Array(2D array=w355) -> (transposed array=w376:dbl[][])
        n125 = for {
          tunnel: w376 -> [w524] mode=indexing
          n126 = global read "9213通道配置全局.vi" "9213通道配置全局"() -> (w523:bool[])
          n127 = call "9229电压-通道配置.vi"("数组"=w523, "数组 2"=w524) -> ("输出簇"=→"9213数据":T6, "通道处理后"=w521:dbl[])  [unwired: 7 in, 1 out]
          n128 = Index Array(array=w521) -> (element #1=→"9213通道1数据":dbl, element #2=→"9213通道2数据":dbl, element #3=→"9213通道3数据":dbl, element #4=→"9213通道4数据":dbl, element #5=→"9213通道5数据":dbl, element #6=→"9213通道6数据":dbl, element #7=→"9213通道7数据":dbl, element #8=→"9213通道8数据":dbl, element #9=→"9213通道9数据":dbl, element #10=→"9213通道10数据":dbl, element #11=→"9213通道11数据":dbl, element #12=→"9213通道12数据":dbl, element #13=→"9213通道13数据":dbl, element #14=→"9213通道14数据":dbl, element #15=→"9213通道15数据":dbl, element #16=→"9213通道16数据":dbl)  [unwired: 16 in]
        }
        n129 = Reciprocal(x=2000.0) -> (1/x=w352:dbl)
        n130 = TCP Read(connection ID=w346, bytes to read=w437, 9:-1 ("超时毫秒(25000)")) -> (connection ID out=w441:refnum<k5>, data out=w438:string, error out=w335:errorcluster)  [unwired: 2 in]
        n131 = Type Cast(type=w437, x=w438) -> (*(type *) &x=w439:i32)
        n132 = TCP Read(connection ID=w441, bytes to read=w439) -> (connection ID out=w434:refnum<k5>, data out=w436:string, error out=w324:errorcluster)  [unwired: 3 in]
        n133 = Type Cast(type=dbl[] [], x=w436) -> (*(type *) &x=w359:dbl[])
        n134 = Decimate 1D Array(w359) -> (w360:dbl[], w361:dbl[], w362:dbl[], w363:dbl[], w364:dbl[], w365:dbl[], w366:dbl[], w367:dbl[], w368:dbl[], w369:dbl[], w370:dbl[], w371:dbl[], w372:dbl[], w373:dbl[], w374:dbl[], w375:dbl[])
        n135 = Build Array(w360, w361, w362, w363, w364, w365, w366, w367, w368, w369, w370, w371, w372, w373, w374, w375) -> (w354:dbl[][])
        n136 = for {
          tunnel: [w460] -> w330 mode=indexing
          tunnel: w354 -> [w459] mode=indexing
          tunnel: w353 -> [w458]
          tunnel: w352 -> [w457]
          n137 = Bundle By Name("Y"=w459, "t0"=w458, "dt"=w457) -> (w460:waveform(dbl))  [unwired: 1 in]
        }
        n138 = call "数据存储-9229.vi"("错误输入（无错误）"=w341, "9229数据"=w330, "tdms文件输入"=w342) -> ("错误输出"=w339:errorcluster, "tdms文件输出"=w340:refnum<k34>)  [unwired: 7 in]
        n139 = Transpose 2D Array(2D array=w354) -> (transposed array=w358:dbl[][])
        n140 = for {
          tunnel: w358 -> [w544] mode=indexing
          n141 = global read "9229通道配置全局.vi" "9229通道配置全局"() -> (w543:bool[])
          n142 = call "9229电压-通道配置.vi"("数组"=w543, "数组 2"=w544) -> ("输出簇"=→"9229":T6, "通道处理后"=w541:dbl[])  [unwired: 7 in, 1 out]
          n143 = Index Array(array=w541) -> (element #1=→"9229通道1数据":dbl, element #2=→"9229通道2数据":dbl, element #3=→"9229通道3数据":dbl, element #4=→"9229通道4数据":dbl, element #5=→"9229通道5数据":dbl, element #6=→"9229通道6数据":dbl, element #7=→"9229通道7数据":dbl, element #8=→"9229通道8数据":dbl, element #9=→"9229通道9数据":dbl, element #10=→"9229通道10数据":dbl, element #11=→"9229通道11数据":dbl, element #12=→"9229通道12数据":dbl, element #13=→"9229通道13数据":dbl, element #14=→"9229通道14数据":dbl, element #15=→"9229通道15数据":dbl, element #16=→"9229通道16数据":dbl)  [unwired: 16 in]
        }
        n144 = Get Date/Time In Seconds() -> (seconds since 1Jan1904=w350:timestamp)
        n145 = Reciprocal(x=1000.0) -> (1/x=w349:dbl)
        n146 = TCP Read(connection ID=w434, bytes to read=w430, 9:-1 ("超时毫秒(25000)")) -> (connection ID out=w433:refnum<k5>, data out=w431:string, error out=w334:errorcluster)  [unwired: 2 in]
        n147 = Type Cast(type=w430, x=w431) -> (*(type *) &x=w429:i32)
        n148 = TCP Read(connection ID=w433, bytes to read=w429) -> (data out=w428:string, error out=w323:errorcluster)  [unwired: 3 in, 1 out]
        n149 = Type Cast(type=dbl[] [], x=w428) -> (*(type *) &x=w426:dbl[])
        n150 = Decimate 1D Array(w426) -> (w425:dbl[], w424:dbl[], w423:dbl[], w422:dbl[], w421:dbl[], w420:dbl[], w419:dbl[], w418:dbl[], w417:dbl[], w416:dbl[], w415:dbl[], w414:dbl[], w413:dbl[], w412:dbl[], w411:dbl[], w410:dbl[], w409:dbl[], w408:dbl[], w407:dbl[], w406:dbl[], w405:dbl[], w404:dbl[], w403:dbl[], w402:dbl[], w401:dbl[], w400:dbl[], w399:dbl[], w398:dbl[], w397:dbl[], w396:dbl[], w395:dbl[], w394:dbl[])
        n151 = Build Array(w425, w424, w423, w422, w421, w420, w419, w418, w417, w416, w415, w414, w413, w412, w411, w410, w409, w408, w407, w406, w405, w404, w403, w402, w401) -> (w351:dbl[][])
        n152 = Transpose 2D Array(2D array=w351) -> (transposed array=w356:dbl[][])
        n153 = for {
          tunnel: w356 -> [w504] mode=indexing
          n154 = global read "9205电压通道配置全局.vi" "9205电压通道配置全局"() -> (w503:bool[])
          n155 = call "9205电压-通道配置.vi"("输入值数组"=w504, "9205通道配置数组"=w503) -> ("输出簇"=→"9205电压":T7, "通道处理后的数组"=w501:dbl[])  [unwired: 7 in, 1 out]
          n156 = Index Array(array=w501) -> (element #1=→"9205电压通道1":dbl, element #2=→"9205电压通道2":dbl, element #3=→"9205电压通道3":dbl, element #4=→"9205电压通道4":dbl, element #5=→"9205电压通道5":dbl, element #6=→"9205电压通道6":dbl, element #7=→"9205电压通道7":dbl, element #8=→"9205电压通道8":dbl, element #9=→"9205电压通道9":dbl, element #10=→"9205电压通道10":dbl, element #11=→"9205电压通道11":dbl, element #12=→"9205电压通道12":dbl, element #13=→"9205电压通道13":dbl, element #14=→"9205电压通道14":dbl, element #15=→"9205电压通道15":dbl, element #16=→"9205电压通道16":dbl, element #17=→"9205电压通道17":dbl, element #18=→"9205电压通道18":dbl, element #19=→"9205电压通道19":dbl, element #20=→"9205电压通道20":dbl, element #21=→"9205电压通道21":dbl, element #22=→"9205电压通道22":dbl, element #23=→"9205电压通道23":dbl, element #24=→"9205电压通道24":dbl, element #25=→"9205电压通道25":dbl)  [unwired: 25 in]
        }
        n157 = for {
          tunnel: [w456] -> w329 mode=indexing
          tunnel: w351 -> [w455] mode=indexing
          tunnel: w350 -> [w454]
          tunnel: w349 -> [w453]
          n158 = Bundle By Name("Y"=w455, "t0"=w454, "dt"=w453) -> (w456:waveform(dbl))  [unwired: 1 in]
        }
        n159 = call "数据存储-9205电压.vi"("错误输入（无错误）"=w339, "9205电压数据"=w329, "tdms文件输入"=w340) -> ("错误输出"=w337:errorcluster, "tdms文件输出"=w338:refnum<k34>)  [unwired: 7 in]
        n160 = Build Array(w400, w399, w398, w397, w396, w395, w394) -> (w348:dbl[][])
        n161 = Transpose 2D Array(2D array=w348) -> (transposed array=w357:dbl[][])
        n162 = for {
          tunnel: w357 -> [w475] mode=indexing
          n163 = global read "9205电流通道配置全局.vi" "9205电流通道配置全局"() -> (w474:bool[])
          n164 = call "9205电流-通道配置.vi"("输入数组"=w475, "9205电流通道数组"=w474) -> ("输出簇"=→"9205电流 2":cluster{dbl, dbl, dbl, dbl, dbl, dbl, dbl}, "通道处理后的数组"=w472:dbl[])  [unwired: 7 in, 1 out]
          n165 = Index Array(array=w472) -> (element #1=→"9205电流通道1":dbl, element #2=→"9205电流通道2":dbl, element #3=→"9205电流通道3":dbl, element #4=→"9205电流通道4":dbl, element #5=→"9205电流通道5":dbl, element #6=→"9205电流通道6":dbl, element #7=→"9205电流通道7":dbl)  [unwired: 7 in]
        }
        n166 = for {
          tunnel: [w452] -> w328 mode=indexing
          tunnel: w350 -> [w451]
          tunnel: w349 -> [w450]
          tunnel: w348 -> [w449] mode=indexing
          n167 = Bundle By Name("Y"=w449, "t0"=w451, "dt"=w450) -> (w452:waveform(dbl))  [unwired: 1 in]
        }
        n168 = call "数据存储-9205电流.vi"("错误输入（无错误）"=w337, "9205电流数据"=w328, "tdms文件输入"=w338) -> ("错误输出"=w326:errorcluster, "tdms文件输出"=w327:refnum<k34>)  [unwired: 7 in]
      }
    }
    n169 = Compound Arithmetic op=OR(w312, w311, w310, w315, w316, w318, w319) -> (w317:bool)
  }
  n170 = Obtain Queue(name (unnamed)="UImessage" ("名称（未命名）"), element data type=T9 {"message"="", "变体数据"=variant} ("命令消息")) -> (queue out=w94:refnum<queue>, error out=w95:errorcluster)  [unwired: 3 in, 1 out]
  n171 = register-events(error in=w7, w4) -> (reference out=w8:refnum<event-registration>)  [unwired: 1 in, 1 out]
  n172 = while {
    tunnel: w3 -> [_]
    tunnel: w8 -> [w550]
    tunnel: [w549] -> w6
    tunnel: w94 -> [w552]
    tunnel: w95 -> [w551]
    tunnel: [w548] -> _
    stop <- w547 stop-if-true
    n173 = event shown="[2] \"触发采集\": 鼠标按下" {
      selector: w550 -> [_ _ _ _ _ _ _]
      dyn-events: [_ _ _ _ _ _ _] -> w549
      timeout: _ -> [_ _ _ _ _ _ _]
      tunnel: w552 -> [w560 w567 w576 w583 w593 w600 _]
      tunnel: [w560 w566 w575 w581 w591 w598 _] -> w545
      tunnel: w551 -> [w559 w565 w574 w582 w592 w599 _]
      tunnel: [w559 w564 w573 w580 w590 w597 _] -> w548
      tunnel: [_ _ _ _ _ _ TRUE] -> w546
      event Timeout {
        n174 = event-data() -> ()  [unwired: 1 in, 3 out]
      }
      event "退出": Value Change {
        n175 = event-data() -> ()  [unwired: 1 in, 6 out]
        n176 = Bundle By Name(cluster=T9 {"message"="", "变体数据"=variant} ("命令消息"), "message"="退出") -> (w561:T9)
        n177 = Enqueue Element(queue=w567, element=w561, error in (no error)=w565) -> (queue out=w566:refnum<queue>, error out=w564:errorcluster)  [unwired: 1 in, 1 out]
      }
      event "触发采集": Mouse Down {
        n178 = event-data() -> ()  [unwired: 1 in, 8 out]
        n179 = To Variant(anything="配置簇") -> (Variant=w569:variant)
        n180 = Bundle By Name(cluster=T9 {"message"="", "变体数据"=variant} ("命令消息"), "message"="开始采集", "变体数据"=w569) -> (w570:T9)
        n181 = Enqueue Element(queue=w576, element=w570, error in (no error)=w574) -> (queue out=w575:refnum<queue>, error out=w573:errorcluster)  [unwired: 1 in, 1 out]
      }
      event "连接": Value Change {
        n182 = event-data() -> ()  [unwired: 1 in, 6 out]
        n183 = Bundle By Name(cluster=T9 {"message"="", "变体数据"=variant} ("命令消息"), "message"="连接") -> (w577:T9)
        n184 = Enqueue Element(queue=w583, element=w577, error in (no error)=w582) -> (queue out=w581:refnum<queue>, error out=w580:errorcluster)  [unwired: 1 in, 1 out]
      }
      event "发送数据到UI": Mouse Down {
        n185 = event-data() -> ()  [unwired: 1 in, 8 out]
        n186 = control-ref of="配置簇"() -> (w584:refnum<vi>)
        n187 = property class="Clust (严格)"(reference=w584) -> ("Value"=w589:T4)  [unwired: 1 in, 2 out]
        n188 = To Variant(anything=w589) -> (Variant=w587:variant)
        n189 = Bundle By Name(cluster=T9 {"message"="", "变体数据"=variant} ("命令消息"), "message"="初始化", "变体数据"=w587) -> (w585:T9)
        n190 = Enqueue Element(queue=w593, element=w585, error in (no error)=w592) -> (queue out=w591:refnum<queue>, error out=w590:errorcluster)  [unwired: 1 in, 1 out]
      }
      event "停止发送数据到UI": Value Change {
        n191 = event-data() -> ()  [unwired: 1 in, 6 out]
        n192 = Bundle By Name(cluster=T9 {"message"="", "变体数据"=variant} ("命令消息"), "message"="停止采集") -> (w594:T9)
        n193 = Enqueue Element(queue=w600, element=w594, error in (no error)=w599) -> (queue out=w598:refnum<queue>, error out=w597:errorcluster)  [unwired: 1 in, 1 out]
      }
      event User Event {
        n194 = event-data() -> ()  [unwired: 1 in, 5 out]
      }
    }
    n195 = case shown="无错误" w548 {
      tunnel: [w553 TRUE] -> w547
      tunnel: w546 -> [w553 _]
      tunnel: w545 -> [_ w557]
      frame No Error {
      }
      frame Error {
        n196 = Bundle By Name(cluster=T9 {"message"="", "变体数据"=variant} ("命令消息"), "message"="退出") -> (w554:T9)
        n197 = Enqueue Element(queue=w557, element=w554) -> ()  [unwired: 2 in, 3 out]
      }
    }
  }
  n198 = while {
    tunnel: w94 -> [w608]
    tunnel: w4 -> [w602]
    stop <- w603 stop-if-true
    n199 = Dequeue Element(queue=w608) -> (queue out=w607:refnum<queue>, element=w604:T9, error out=w606:errorcluster)  [unwired: 2 in, 1 out]
    n200 = Unbundle By Name(w604) -> ("message"=w605:string)
    "UI命令" <- w605
    n201 = case shown="\"初始化\", \"开始采集\", \"停止采集\"" w605 {
      tunnel: w607 -> [_ w610 w630 _ _]
      tunnel: w606 -> [_ w609 w629 _ _]
      tunnel: w604 -> [_ _ _ _ w656]
      tunnel: [_ w612 _ _ _] -> w603
      tunnel: w602 -> [_ w611 _ _ _]
      frame Default {
      }
      frame "退出" {
        n202 = flat-sequence {
          tunnel: [w617] -> w612
          tunnel: w611 -> [w616]
          tunnel: w610 -> [w614]
          tunnel: w609 -> [w613]
          frame #0 {
            w617 = TRUE ("UIdata停止")
            n203 = Generate User Event(user event=w616, event data cluster=TRUE ("事件数据")) -> ()  [unwired: 2 in, 2 out]
            n204 = global read "UI网络流写入方端点全局.vi" "UI网络流写入方端点全局"() -> (w619:refnum<k21>)
            n205 = global read "UI-TCP-IP连接全局.vi" "UI-TCP/IP连接全局"() -> (w618:refnum<k5>)
            n206 = Release Queue(queue=w614, error in (no error)=w613) -> ()  [unwired: 1 in, 3 out]
            n207 = global write "UI-all停止全局.vi" "UI-all停止"(w617) -> ()
            n208 = TCP Close Connection(connection ID=w618) -> ()  [unwired: 2 in, 2 out]
            n209 = Destroy Stream Endpoint(11:w619) -> ()  [unwired: 1 in, 1 out]
            n210 = local write "连接成功？"(FALSE ("连接成功？")) -> ()
          }
        }
      }
      frame "连接" {
        n211 = Create Network Stream Writer Endpoint(7:500000 ("写入方缓冲大小"), 9:T9 {"message"="", "变体数据"=variant} ("命令消息"), 10:"//169.254.66.100/RT" ("读取方url"), 11:"UI" ("写入方名称")) -> (0:w632:errorcluster, 3:w635:refnum<k21>)  [unwired: 3 in]
        n212 = TCP Open Connection(address="169.254.66.100" ("地址"), remote port or service name=u16 6001 ("远程端口或服务名称"), error in (no error)=w632) -> (connection ID=w631:refnum<k5>, error out=w628:errorcluster)  [unwired: 2 in]
        n213 = case shown="无错误" w628 {
          tunnel: w635 -> [w642 w650]
          tunnel: [w645 refnum<k5> refnum ("connection ID")] -> w623
          tunnel: w631 -> [w645 w649]
          tunnel: w630 -> [_ w653]
          tunnel: w629 -> [_ w652]
          tunnel: [errorcluster {"status"=FALSE, "code"=0, "source"=""} ("error out") w648] -> w626
          tunnel: [errorcluster {"status"=FALSE, "code"=0, "source"=""} ("error out") w647] -> w625
          tunnel: [w642 refnum<k21> refnum ("写入方名称")] -> w621
          frame No Error {
          }
          frame Error {
            n214 = Destroy Stream Endpoint(11:w650) -> (0:w648:errorcluster)  [unwired: 1 in]
            n215 = TCP Close Connection(connection ID=w649) -> (error out=w647:errorcluster)  [unwired: 2 in, 1 out]
            n216 = call "消息数据入队列.vi"("错误输入（无错误）"=w652, "message"="断开UI", "队列输入"=w653) -> ()  [unwired: 7 in, 2 out]
          }
        }
        n217 = Not(x=w628) -> (.not. x?=w627:bool)
        n218 = global write "UI网络流写入方端点全局.vi" "UI网络流写入方端点全局"(w621) -> ()
        n219 = global write "UI-TCP-IP连接全局.vi" "UI-TCP/IP连接全局"(w623) -> ()
        n220 = case shown="真" w627 {
          selector: w627 -> [_ w641]
          tunnel: [T11."Enabled" ("禁用") T11."Disabled and Grayed Out" ("禁用")] -> w624
          tunnel: w626 -> [_ _]
          tunnel: w625 -> [_ _]
          frame False {
          }
          frame True {
            "连接成功？" <- w641
          }
        }
        n221 = property on="连接" class="Bool"("DisabledEnum"=w624) -> ()  [unwired: 2 in, 2 out]
      }
      frame "断开UI" {
        n222 = property on="连接成功？" class="Bool (严格)"("DisabledEnum"=T11."Enabled" ("禁用")) -> ()  [unwired: 2 in, 2 out]
      }
      frame "初始化", "开始采集", "停止采集" {
        n223 = local read "连接成功？"() -> (w657:bool)
        n224 = case shown="真" w657 {
          tunnel: w656 -> [_ w659]
          frame False {
          }
          frame True {
            n225 = global read "UI网络流写入方端点全局.vi" "UI网络流写入方端点全局"() -> (w658:refnum<k21>)
            n226 = shared-variable-write(w658, w659) -> ()  [unwired: 2 in, 3 out]
          }
        }
      }
    }
  }
  n227 = Unregister For Events(event registration refnum=w6) -> (error out=w5:errorcluster)  [unwired: 1 in]
  n228 = Destroy User Event(user event=w4, error in=w5) -> ()  [unwired: 1 out]
  n229 = TDMS Close(8:w1, 11:w2) -> ()  [unwired: 2 out]
